vi "ejer3.vi"() -> ()   [LabVIEW 2014]
panel:
  in  "Frecuencia":dbl
  in  "Voltaje - Amplitud":dbl
  in  "?":bool
  out "Potencia":dbl(knob) scale=0.0..75.0
  in  "Resistencia":dbl(knob) scale=0.0..200.0
  out "Gráfica":dynamicdata(graph)
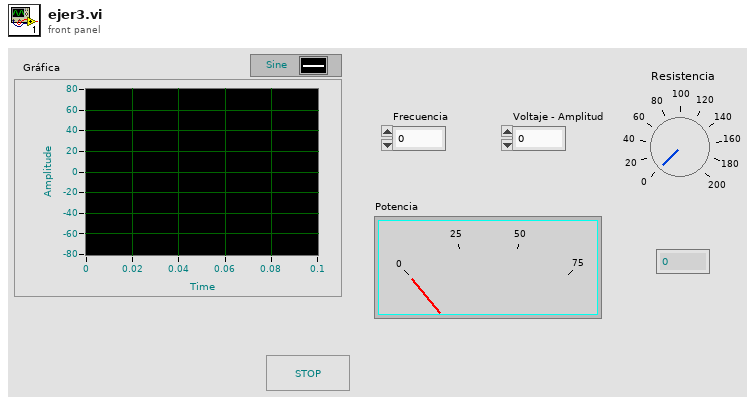
[diagram p1: front panel]
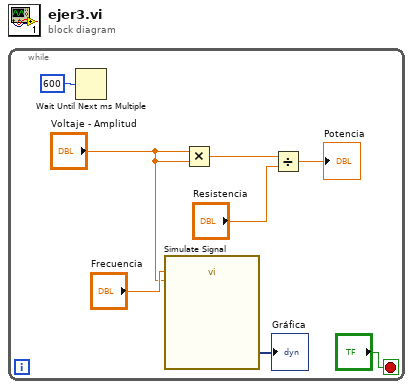
[diagram p0: block diagram]
diagram:
  n1 = while {
    stop <- "?" stop-if-true
    n2 = Wait Until Next ms Multiple(millisecond multiple=600) -> ()  [unwired: 1 out]
    n3 = call "Simulate Signal"("Frequency"="Frecuencia", "Amplitude"="Voltaje - Amplitud") -> ("Sine"=→"Gráfica":dynamicdata)  [unwired: 12 in, 1 out]
    n4 = Multiply(x="Voltaje - Amplitud", y="Voltaje - Amplitud") -> (x*y=w5:dbl)
    n5 = Divide(x=w5, y="Resistencia") -> (x/y=→"Potencia":dbl)
  }
